vi "Example Simple.vi"() -> ()   [LabVIEW 2013]
uses:
  C:/tf/play/labview/Tinkerforge.dll
panel:
  in  "uid":string="fBk"
  in  "port":i32=4223
  in  "host":string="localhost"
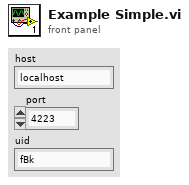
[diagram p1: front panel]
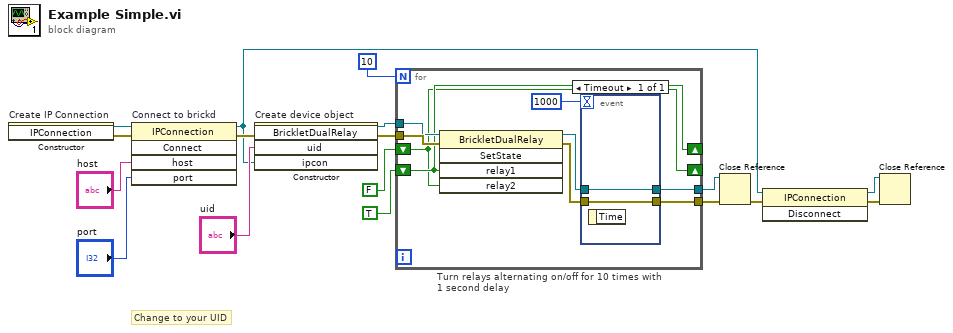
[diagram p0: block diagram]
diagram:
  # "Change to your UID"
  n1 = constructor on="Create IP Connection" class="IPConnection"() -> (reference out=w17:refnum<k24>, error out=w8:errorcluster)  [unwired: 3 in, 1 out]
  n2 = invoke on="Connect to brickd" class="IPConnection" method="Connect"(reference=w17, error in=w8, "host"="host", "port"="port") -> (reference out=w10:refnum<k24>, error out=w13:errorcluster)  [unwired: 1 in, 3 out]
  n3 = constructor on="Create device object" class="BrickletDualRelay"(error in=w13, "uid"="uid", "ipcon"=w10) -> (reference out=w3:refnum<k24>, error out=w4:errorcluster)  [unwired: 2 in, 3 out]
  n4 = for "Turn relays alternating on/off for 10 times with 1 second delay" {
    N: 10 -> [_]
    tunnel: w4 -> [w26]
    tunnel: w3 -> [w25]
    tunnel: [w19] -> w2
    tunnel: [w21] -> w1
    shift-right: [w23] -> _
    shift-left: TRUE -> [w24]
    shift-right: [w24] -> _
    shift-left: FALSE -> [w23]
    n5 = invoke class="BrickletDualRelay" method="SetState"(reference=w25, error in=w26, "relay1"=w24, "relay2"=w23) -> (reference out=w20:refnum<k24>, error out=w18:errorcluster)  [unwired: 1 in, 3 out]
    n6 = event shown="[0] Timeout" {
      selector: _ -> [_]
      dyn-events: _ -> [_]
      timeout: 1000 -> [_]
      tunnel: [w28] -> w21
      tunnel: w20 -> [w28]
      tunnel: [w27] -> w19
      tunnel: w18 -> [w27]
      event Timeout {
        n7 = event-data() -> ()  [unwired: 1 in, 1 out]
      }
    }
  }
  n8 = Close Reference(reference=w1, error in (no error)=w2) -> (error out=w12:errorcluster)
  n9 = invoke class="IPConnection" method="Disconnect"(reference=w10, error in=w12) -> (reference out=w9:refnum<k24>, error out=w11:errorcluster)  [unwired: 1 in, 1 out]
  n10 = Close Reference(reference=w9, error in (no error)=w11) -> ()  [unwired: 1 out]
